vi "Find Class Ancestry.vi"(8 "error in (no error)":errorcluster, 11 "reference in":refnum<vi>) -> (0 "error out":errorcluster, 2 "Class Ancestry":path[](array[path]), 3 "reference out":refnum<vi>)   [LabVIEW 2020, in "Icon Decorator.lvlib" / "Icon Decorator.lvclass"]
uses:
  Icon Decorator.lvclass
  Icon Decorator.lvclass/Icon Decorator.ctl
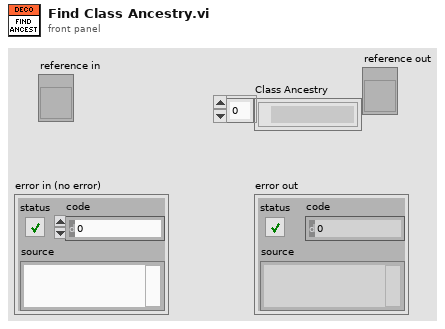
[diagram p1: front panel]
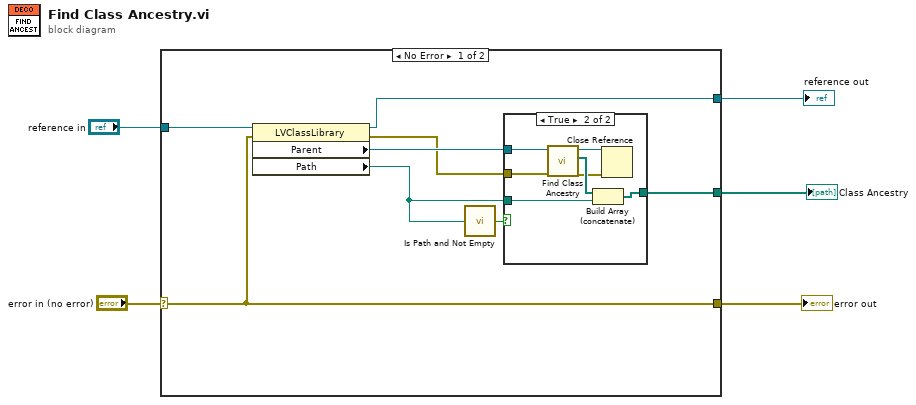
[diagram p0: block diagram]
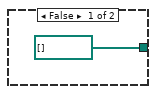
[diagram p2: hidden frame]
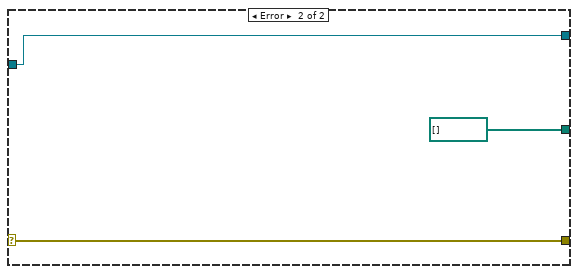
[diagram p3: hidden frame]
diagram:
  n1 = case shown="No Error" "error in (no error)" {
    selector: "error in (no error)" -> [w7 w24]
    tunnel: "reference in" -> [w13 w22]
    tunnel: [w11 path[] [] ("Class Ancestry")] -> w4
    tunnel: [w7 w24] -> w2
    tunnel: [w6 w22] -> w1
    frame No Error {
      n2 = property class="LVClassLibrary"(reference=w13, error in=w7) -> (reference out=w6:refnum<vi>, error out=w10:errorcluster, "Parent"=w12:refnum<vi>, "Path"=w9:path)
      n3 = call <vilib>:"Is Path and Not Empty.vi"("path"=w9) -> ("Is Path and Not Empty?"=w8:bool)  [unwired: 4 in]
      n4 = case shown="True" w8 {
        tunnel: [path[] [] ("Class Ancestry") w20] -> w11
        tunnel: w12 -> [_ w21]
        tunnel: w9 -> [_ w19]
        tunnel: w10 -> [_ w18]
        frame False {
        }
        frame True {
          n5 = call "Find Class Ancestry.vi"("error in (no error)"=w18, "reference in"=w21) -> ("error out"=w15:errorcluster, "Class Ancestry"=w17:path[], "reference out"=w16:refnum<vi>)  [unwired: 7 in]
          n6 = Build Array (concatenate)(w17, w19) -> (w20:path[])
          n7 = Close Reference(reference=w16, error in (no error)=w15) -> ()  [unwired: 1 out]
        }
      }
    }
    frame Error {
    }
  }
  "Class Ancestry" <- w4
  "error out" <- w2
  "reference out" <- w1
